vi "update forms simple tables.vi"(8 "error in (no error)":errorcluster) -> (0 "error out":errorcluster)   [LabVIEW 2020]
uses:
  forms AF/Update Fields Logic/Field FK PK Info.ctl
  forms AF/Autoclose manager/Form ID.ctl
  forms AF/Update Fields Logic Simple Table/Update Fields Logic Simple Table.lvclass
  forms AF/Update Fields Logic/Form FK Fields.ctl
  <vilib>/addons/_JKI Toolkits/Caraya/classes/Assert/Assert Equal Value_Variant.vi
  <vilib>/addons/_JKI Toolkits/Caraya/classes/Test/Test.lvclass
  <vilib>/addons/_JKI Toolkits/Caraya/classes/Assert/Assert.lvclass
  forms AF/Form Server Interfaces.lvlib
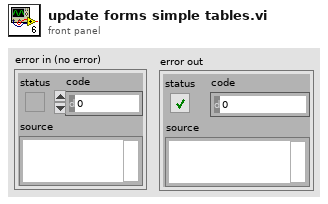
[diagram p1: front panel]
types:
  T1 = typedef "Form Server Interfaces.lvlib/Form FK Fields.ctl" = cluster{"Form IDs":T2[], "Field IDs":string[]}
  T2 = typedef "Form Server Interfaces.lvlib/Form ID.ctl" = cluster{"Name":string, "Panel type":string}
  T3 = typedef "Form Server Interfaces.lvlib/Field FK PK Info.ctl" = cluster{"Field ID":string[], "FK Table":string[], "FK Column":string[], "PK Table":string[], "PK Column":string[]}
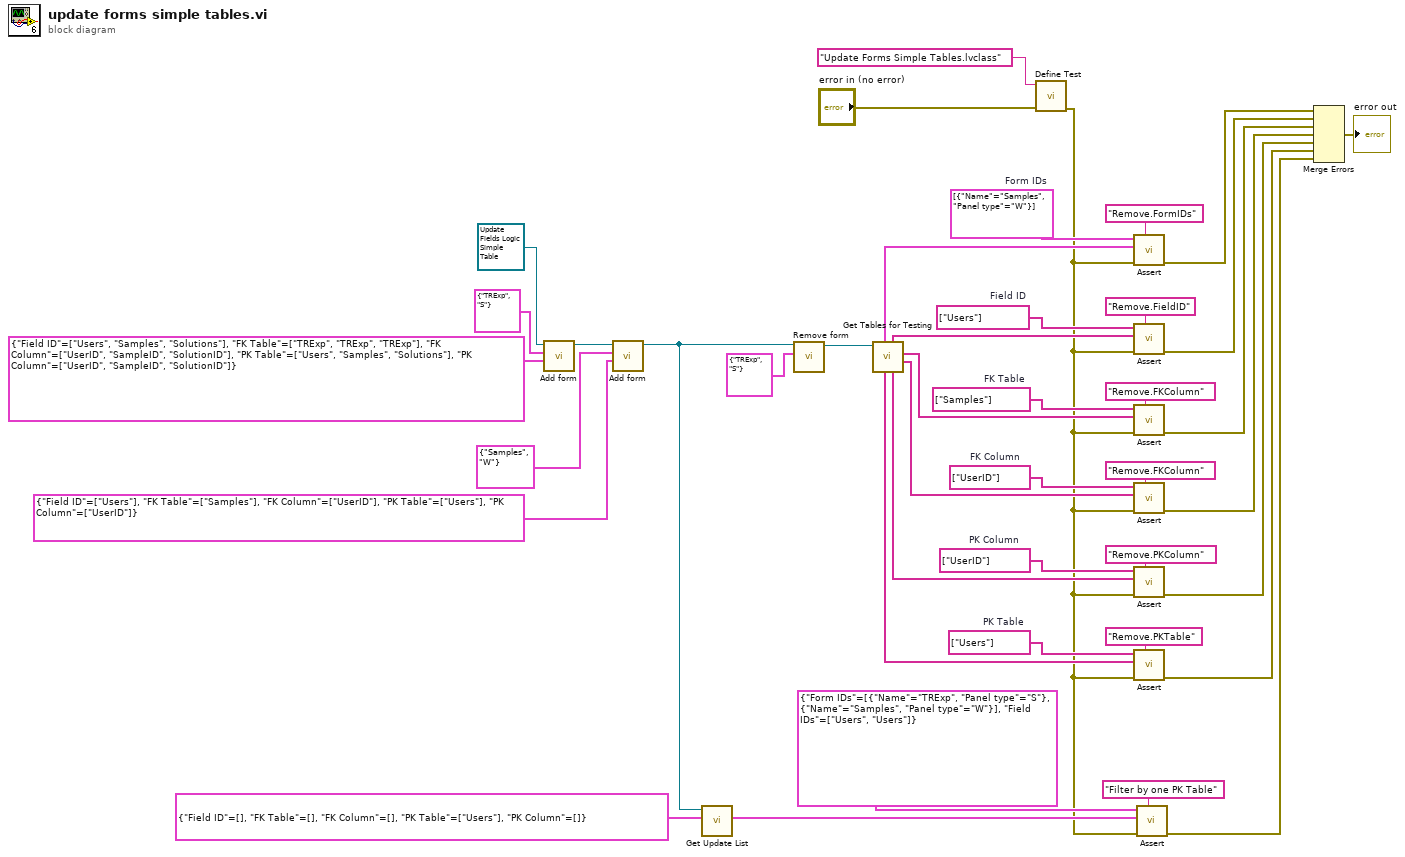
[diagram p0: block diagram]
diagram:
  w23 = string[] ["Users"]  # PK Table
  w25 = string[] ["UserID"]  # PK Column
  w27 = string[] ["UserID"]  # FK Column
  w29 = string[] ["Samples"]  # FK Table
  w31 = string[] ["Users"]  # Field ID
  w33 = T2[] [{"Name"="Samples", "Panel type"="W"}]  # Form IDs
  n1 = call-dynamic "Add form.vi"("FK/PK Info"=T3 {"Field ID"=["Users", "Samples", "Solutions"], "FK Table"=["TRExp", "TRExp", "TRExp"], "FK Column"=["UserID", "SampleID", "SolutionID"], "PK Table"=["Users", "Samples", "Solutions"], "PK Column"=["UserID", "SampleID", "SolutionID"]}, "Form ID"=T2 {"Name"="TRExp", "Panel type"="S"}, "Update Fields Logic Simple Table in"=refnum<class "Update Fields Logic Simple Table.lvclass"> refnum) -> ("Update Fields Logic Simple Table out"=w38:refnum<class "Update Fields Logic Simple Table.lvclass">)  [unwired: 6 in, 2 out]
  n2 = call-dynamic "Add form.vi"("FK/PK Info"=T3 {"Field ID"=["Users"], "FK Table"=["Samples"], "FK Column"=["UserID"], "PK Table"=["Users"], "PK Column"=["UserID"]}, "Form ID"=T2 {"Name"="Samples", "Panel type"="W"}, "Update Fields Logic Simple Table in"=w38) -> ("Update Fields Logic Simple Table out"=w15:refnum<class "Update Fields Logic Simple Table.lvclass">)  [unwired: 6 in, 2 out]
  n3 = call-dynamic "Get Update List.vi"("Filter FK/PK"=T3 {"Field ID"=[], "FK Table"=[], "FK Column"=[], "PK Table"=["Users"], "PK Column"=[]}, "Update Fields Logic Simple Table in"=w15) -> ("Fields to update"=w13:T1)  [unwired: 7 in, 2 out]
  n4 = call-dynamic "Remove form.vi"("Form ID"=T2 {"Name"="TRExp", "Panel type"="S"}, "Update Fields Logic Simple Table in"=w15) -> ("Update Fields Logic Simple Table out"=w35:refnum<class "Update Fields Logic Simple Table.lvclass">)  [unwired: 8 in, 1 out]
  n5 = call "Get Tables for Testing.vi"("Update Fields Logic Simple Table in"=w35) -> ("FK Column"=w28:string[], "FK Table"=w30:string[], "PK Column"=w26:string[], "Field ID"=w32:string[], "PK Table"=w24:string[], "Form IDs"=w34:T2[])  [unwired: 3 in, 2 out]
  n6 = call <vilib>:"Define Test.vi"("error in (no error)"="error in (no error)", "Label (VI Title)"="Update Forms Simple Tables.lvclass") -> ("error out"=w11:errorcluster)  [unwired: 9 in]
  n7 = call-poly <vilib>:"Assert.vi"("Label"="Remove.FormIDs", "error in (no error)"=w11, "Y"=w34, "X"=w33) -> ("error out"=w4:errorcluster)  [unwired: 7 in]
  n8 = call-poly <vilib>:"Assert.vi"("Label"="Remove.FieldID", "error in (no error)"=w11, "Y"=w32, "X"=w31) -> ("error out"=w5:errorcluster)  [unwired: 7 in]
  n9 = call-poly <vilib>:"Assert.vi"("Label"="Remove.FKColumn", "error in (no error)"=w11, "Y"=w30, "X"=w29) -> ("error out"=w6:errorcluster)  [unwired: 7 in]
  n10 = call-poly <vilib>:"Assert.vi"("Label"="Remove.FKColumn", "error in (no error)"=w11, "Y"=w28, "X"=w27) -> ("error out"=w7:errorcluster)  [unwired: 7 in]
  n11 = call-poly <vilib>:"Assert.vi"("Label"="Remove.PKColumn", "error in (no error)"=w11, "Y"=w26, "X"=w25) -> ("error out"=w8:errorcluster)  [unwired: 7 in]
  n12 = call-poly <vilib>:"Assert.vi"("Label"="Remove.PKTable", "error in (no error)"=w11, "Y"=w24, "X"=w23) -> ("error out"=w9:errorcluster)  [unwired: 7 in]
  n13 = call-poly <vilib>:"Assert.vi"("Label"="Filter by one PK Table", "error in (no error)"=w11, "Y"=w13, "X"=T1 {"Form IDs"=[{"Name"="TRExp", "Panel type"="S"}, {"Name"="Samples", "Panel type"="W"}], "Field IDs"=["Users", "Users"]} ("Fields to update")) -> ("error out"=w10:errorcluster)  [unwired: 7 in]
  n14 = Merge Errors(w4, w5, w6, w7, w8, w9, w10) -> (→"error out":errorcluster)
